vi "S2C_5190CR_Poly_SetOutput.vi"(8 "Error In":errorcluster, 10 "Set Output":T1={"OutletPlug"=1, "OutletState"=TRUE, "PowerOnDelay(ms)"=50, "PowerOffDelay(ms)"=0, "WaitOnState"=TRUE, "Timeout(ms)"=10000} {"OutletPlug" items=["Outlet 1"=1, "Outlet 2"=2, "Outlet 3"=3, "Outlet 4"=4, "Outlet 5"=5, "Outlet 6"=6, "Outlet 7"=7, "Outlet 8"=8]}, 11 "Settings":T2={"Driver"="5190CR", "Command"="Set Output", "Return"="ErrorStatus", "Parameters"="", "Timeout"=10.0}) -> (0 "Error Out":errorcluster, 3 "Response":string)   [LabVIEW 2015]
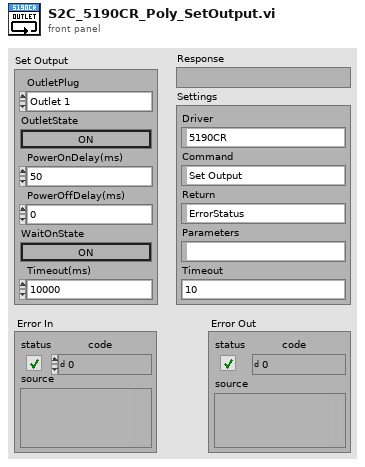
[diagram p1: front panel]
types:
  T1 = cluster{"OutletPlug":u16, "OutletState":bool, "PowerOnDelay(ms)":u32, "PowerOffDelay(ms)":u32, "WaitOnState":bool, "Timeout(ms)":i32}
  T2 = cluster{"Driver":string, "Command":string, "Return":string, "Parameters":string, "Timeout":dbl}
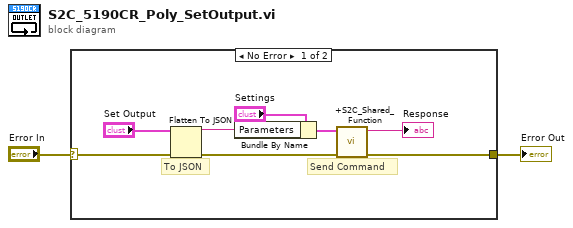
[diagram p0: block diagram]
diagram:
  n1 = case shown="No Error" "Error In" {
    selector: "Error In" -> [w6 w11]
    tunnel: [w5 w11] -> w1
    frame No Error {
      # "To JSON"
      # "Send Command"
      n2 = Flatten To JSON(anything="Set Output", error in (no error)=w6) -> (JSON string=w7:string, 11:w9:errorcluster)  [unwired: 1 in]
      n3 = Bundle By Name(cluster="Settings", "Parameters"=w7) -> (w10:T2)
      n4 = call "+S2C_Shared_Function.vi"("Error In"=w9, "Settings"=w10) -> ("Error Out"=w5:errorcluster, "Response"=→"Response":string)  [unwired: 8 in]
    }
    frame Error {
    }
  }
  "Error Out" <- w1
